vi "UnpackRobotCommandsUDP.vi"(0 "Received String":string="1500,1500") -> (1 "Left Motor Power":i32, 2 "Right Motor Power":i32)   [LabVIEW 2012]
panel:
  out "Robot ID":string
  out "substring after match":string
  out "substring before match":string
  # "Ranges from 1150 to 1750"
  # "or maybe 1000 to 2000"
  # "$,R,1500,1500,S,14,58,555\\r"
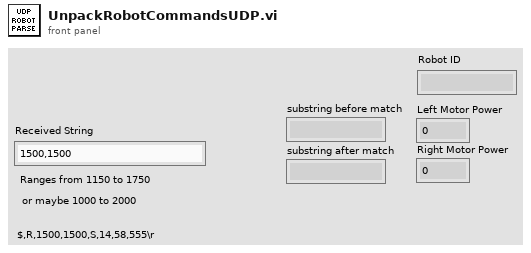
[diagram p1: front panel]
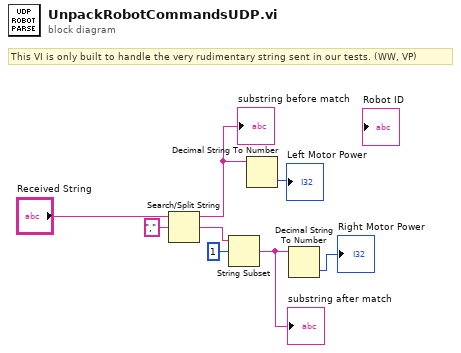
[diagram p0: block diagram]
diagram:
  # "This VI is only built to handle the very rudimentary string sent in our tests. (WW, VP)"
  n1 = Search/Split String(string="Received String", search string/char (-)=",") -> (substring before match=w4:string, match + rest of string=w6:string)  [unwired: 1 in, 1 out]
  "substring before match" <- w4
  n2 = String Subset(string=w6, offset (0)=1) -> (substring=w3:string)  [unwired: 1 in]
  "substring after match" <- w3
  n3 = Decimal String To Number(string=w4) -> (number=→"Left Motor Power":i32)  [unwired: 2 in, 1 out]
  n4 = Decimal String To Number(string=w3) -> (number=→"Right Motor Power":i32)  [unwired: 2 in, 1 out]
